vi "Client RX Loop.vi"(8 "error in (no error)":errorcluster, 11 "TCPMessaging in":refnum<class "TCPMessaging.lvclass">) -> (0 "error out":errorcluster)   [LabVIEW 2020, in "Vecto.lvlib" / "TCPMessaging.lvclass"]
uses:
  TCPMessaging.lvclass
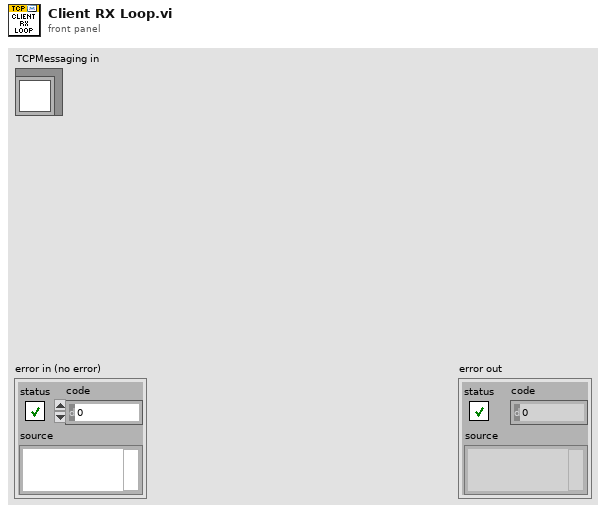
[diagram p1: front panel]
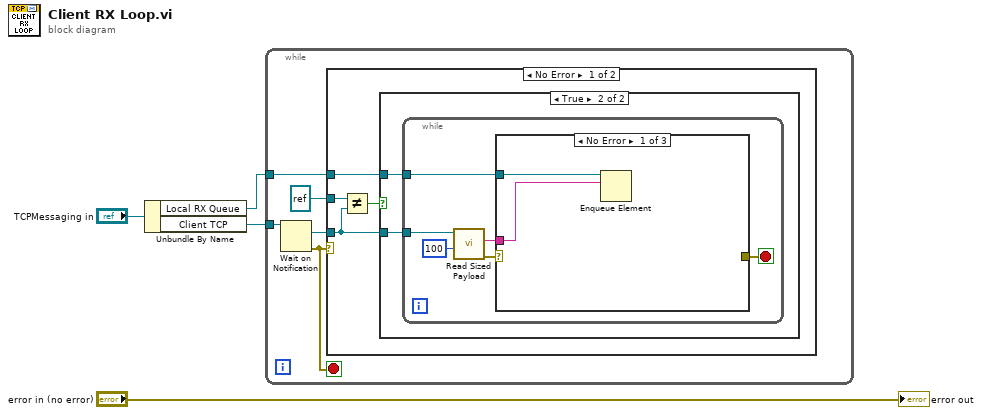
[diagram p0: block diagram]
diagram:
  n1 = Unbundle By Name("TCPMessaging in") -> ("Local RX Queue"=w1:refnum<queue>, "Client TCP"=w2:refnum<notifier>)
  n2 = while {
    tunnel: w2 -> [w9]
    tunnel: w1 -> [w5]
    stop <- w7 stop-if-true
    n3 = Wait on Notification(notifier=w9) -> (notification=w8:refnum<k5>, error out=w7:errorcluster)  [unwired: 3 in, 2 out]
    n4 = case shown="No Error" w7 {
      tunnel: w8 -> [w11 _]
      tunnel: refnum<k5> refnum ("x") -> [w13 _]
      tunnel: w5 -> [w10 _]
      frame No Error {
        n5 = Not Equal?(x=w13, y=w11) -> (x != y?=w12:bool)
        n6 = case shown="True" w12 {
          tunnel: w11 -> [_ w15]
          tunnel: w10 -> [_ w14]
          frame False {
          }
          frame True {
            n7 = while {
              tunnel: w15 -> [w20]
              tunnel: w14 -> [w21]
              stop <- w16 stop-if-true
              n8 = call "Read Sized Payload.vi"("timeout ms (100)"=100, "TCP in"=w20) -> ("error out"=w18:errorcluster, "Payload"=w17:string)  [unwired: 7 in, 1 out]
              n9 = case shown="No Error" w18 {
                selector: w18 -> [_ _ w24]
                tunnel: w21 -> [w23 _ _]
                tunnel: w17 -> [w22 _ _]
                tunnel: [_ _ w24] -> w16
                frame No Error {
                  n10 = Enqueue Element(queue=w23, element=w22) -> ()  [unwired: 2 in, 3 out]
                }
                frame Error {
                }
                frame Default {
                }
              }
            }
          }
        }
      }
      frame Error {
        # "Notifier has been released, shutting down."
      }
    }
  }
  "error out" <- "error in (no error)"
